vi "Read Core OOB RX.vi"(8 "error in (no error)":errorcluster, 11 "CIFCorePlugin in":refnum<class "CIFCorePlugin.lvclass">) -> (0 "error out":errorcluster, 3 "CIFCorePlugin out":refnum<class "CIFCorePlugin.lvclass">)   [LabVIEW 2021, in "CIFCorePlugin.lvclass"]
uses:
  CIFCorePlugin.lvclass
  Typedef/gRPC to Main Command Payload.ctl
  Typedef/gRPC to Main Commands.ctl
  <vilib>/CIF Foundation/CIF CIPC/TypeDefs/Read Configuration.ctl
  <vilib>/CIF Foundation/CIF CIPC/TypeDefs/Read Position.ctl
  CIFCorePlugin.lvclass/CIFCorePlugin.ctl
  Common/Typedef/Plugin State.ctl
  Typedef/Energized States.ctl
  <vilib>/CIF Foundation/CIF Channels Core/ChannelCommon/typedef/New FIFO Instance Response.ctl
  Channels/CIFChannelMng/CIFChannelMng.lvclass/CIFChannelMng.ctl
  <vilib>/CIF Foundation/CIF Channels Core/CIFChannels/CIFChannels.lvclass/CIFChannels.ctl
  a31a91a9-4107-4750-8e0d-44486e9a3a34.vi
  Channels/CIFChannelMng/Core/Send Channel List Update.vi/463ebf4c-8748-40f9-8ad3-9e61c16a01a6.vi
  Channels/CIFChannelMng/Utilities/Get Channel Index by Name.vi
  <vilib>/CIF Foundation/CIF Channels Core/CIFChannels/Accessors/Read Channel State.vi
  <vilib>/CIF Foundation/CIF Channels Core/CIFChannels/Accessors/Read Tag Forced.vi
  Channels/CIFChannelMng/SubVIs/Add Error Channel Manager.vi
  Channels/CIFChannelMng/Core/Send Publisher Instance Return.vi/9db40550-ae0b-4108-a32d-02e81b824dbe.vi
  Channels/CIFChannelMng/SubVIs/Get Original FIFO Channel Name.vi
  <vilib>/CIF Foundation/CIF CIPC/SubVIs/Wait For N Elements Available.vi
  <vilib>/CIF Foundation/CIF CIPC/SubVIs/Check Error.vi
  <vilib>/CIF Foundation/CIF CIPC/SubVIs/Get dll Path.vi
  <vilib>/CIF Foundation/CIF CIPC/SubVIs/Get Element Read Position.vi
  <vilib>/CIF Foundation/CIF CIPC/SubVIs/Set Element Read Position.vi
  <vilib>/CIF Foundation/CIF CIPC/SubVIs/Notify Of New Write.vi
  <vilib>/CIF Foundation/CIF CIPC/SubVIs/Get Element Write Position.vi
  <vilib>/CIF Foundation/CIF Channels Core/ChannelCommon/Utilities/Add Error.vi
  <vilib>/CIF Foundation/CIF Utilities/Errors/Append Error Location.vi
  <vilib>/CIF Foundation/CIF CIPC/SubVIs/Get Element Info Variant.vi
  <vilib>/CIF Foundation/CIF CIPC/SubVIs/Check Error Core.vi
  <vilib>/CIF Foundation/CIF Channels Core/ChannelCommon/Utilities/Add Error Core.vi
  <vilib>/CIF Foundation/CIF Channels Core/CIFChannels/Core/Set Force.vi
  <vilib>/CIF Foundation/CIF Channels Core/CIFChannels/CIFChannels.lvclass
  Channels/CIFChannelMng/CIFChannelMng.lvclass
  <vilib>/CIF Foundation/CIF CIPC/CIF_NI_CIPC.lvlib
  <vilib>/CIF Foundation/CIF Channels Core/ChannelCommon/ChannelCommon.lvlib
  Common/CIFCoreCommon.lvlib
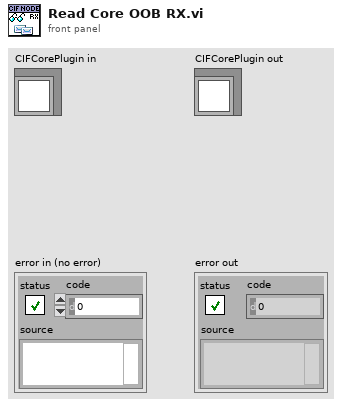
[diagram p1: front panel]
types:
  T1 = typedef "CIFCorePlugin.lvclass/gRPC to Main Command Payload.ctl" = cluster{"OOB_Rx Command":T2, "Array Index":i16}
  T2 = typedef "CIFCorePlugin.lvclass/gRPC to Main Commands.ctl" = enum8{"Start", "Pause", "Stop", "RefreshStats", "UpdateConfig", "Update Clock Map", "Connect Channel", "Force Channel", "Add Publisher Instance", "Remove Publisher Instance", "Prepare"}
  T3 = typedef "CIF_NI_CIPC.lvlib/Read Configuration.ctl" = cluster{"Read Position":T4, "Element Offset":i32, "Prepend Array Size":bool, "Get Read Position":bool}
  T4 = typedef "CIF_NI_CIPC.lvlib/Read Position.ctl" = enum8{"Next", "Newest", "Oldest", "Next Available", "Absolute"}
  T5 = typedef "CIFCoreCommon.lvlib/Plugin State.ctl" = enum8{"Null", "Creating", "Listening", "Running", "CleaningUp", "Destroying", "Prepared", "FTE_Run"}
  T6 = typedef "CIFCorePlugin.lvclass/Energized States.ctl" = enum16{"Listen", "Prepare", "Execute", "Housekeep", "Cleanup", "Destroy"}
  T7 = typedef "ChannelCommon.lvlib/New FIFO Instance Response.ctl" = cluster{"Publisher":string, "Custom Data":u8[]}
  T8 = typedef "Time_CIF_U.lvlib/Clock Conversion Map.ctl" = map{u8, cluster{"Last Reset":i64, "Offset Pair":T9, "Slope":dbl, "1/Slope":dbl}}
  T9 = typedef "Time_CIF_U.lvlib/Timestamp Pair.ctl" = cluster{"System Time":i64, "External Time":i64}
  T10 = typedef "CIFCoreCommon.lvlib/Channel Connection Data.ctl" = cluster{"Publisher Name":string, "Subscriber Name":string, "Connection Data":u8[]}
  T11 = typedef "CIFCoreCommon.lvlib/Channel Force Data.ctl" = cluster{"Channel Name":string, "Force Data":u8[], "Force Active":bool}
  T12 = typedef "CIFCoreCommon.lvlib/FIFO Publisher.ctl" = cluster{"Publisher Name":string, "New FIFO Instance Config":T13}
  T13 = typedef "ChannelCommon.lvlib/New FIFO Instance Configuration.ctl" = cluster{"Backpressure":bool, "Bytes/Message Override":u32, "Messages/FIFO Override":u32, "Custom Data":u8[]}
  T14 = typedef "CIFChannelMng.lvclass/FIFO Publisher Return.ctl" = cluster{"FIFO Instance Config":T7, "error":errorcluster, "Added":bool}
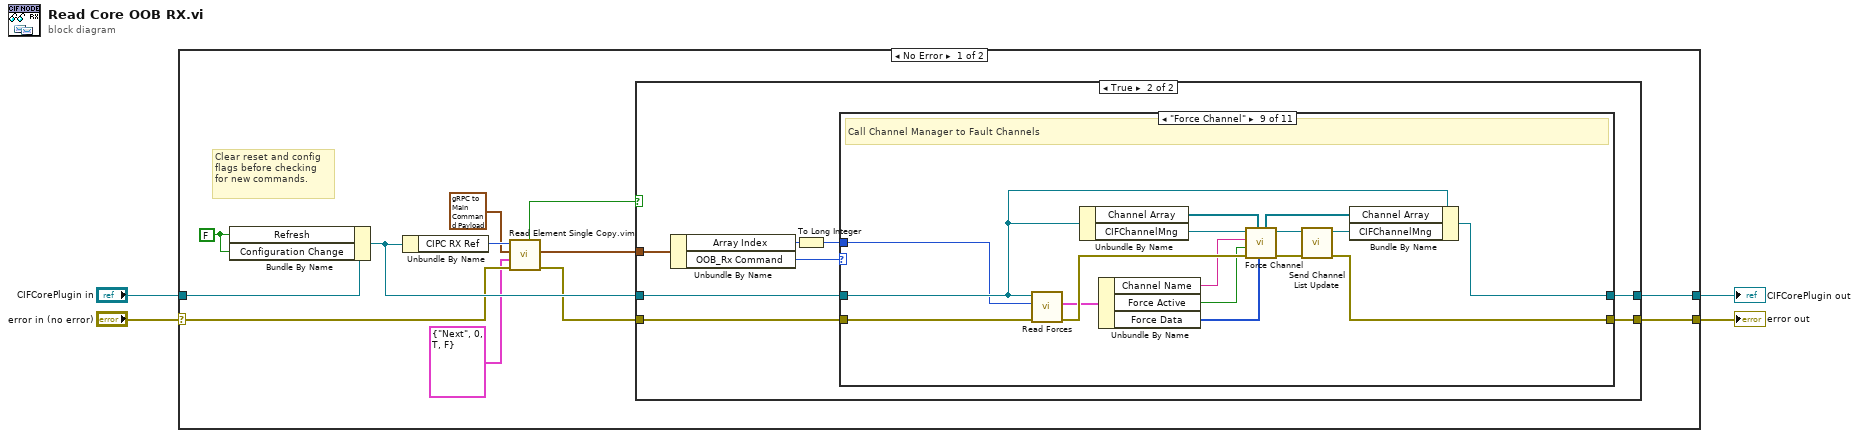
[diagram p0: block diagram]
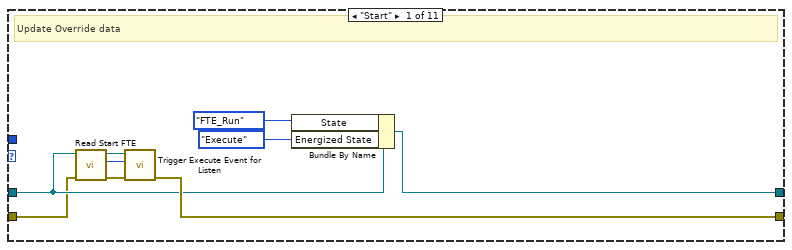
[diagram p3: hidden frame]
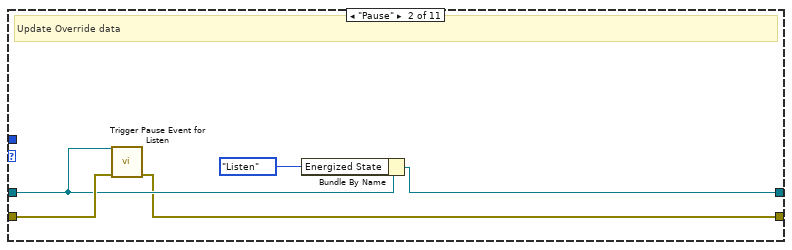
[diagram p4: hidden frame]
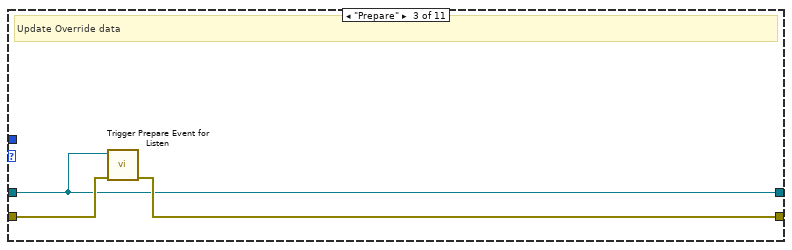
[diagram p5: hidden frame]
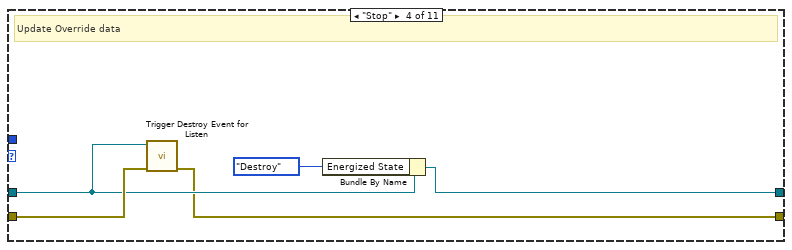
[diagram p6: hidden frame]
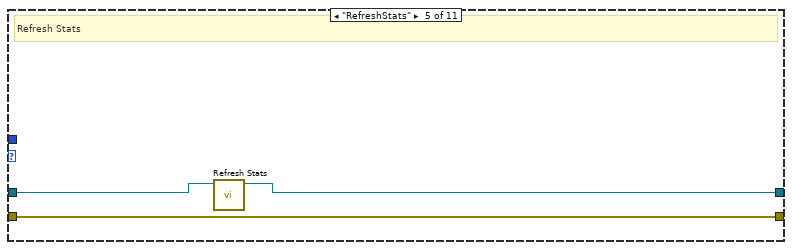
[diagram p7: hidden frame]
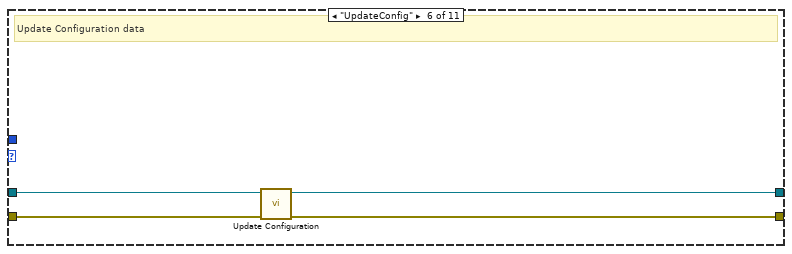
[diagram p8: hidden frame]
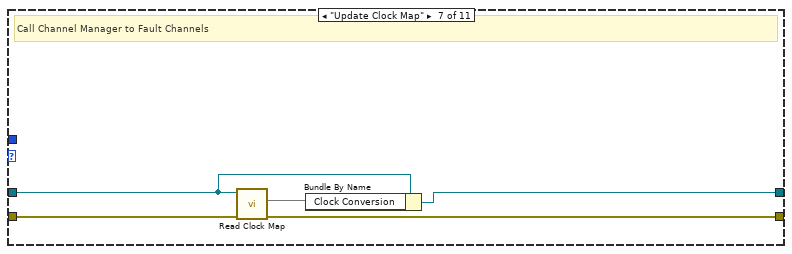
[diagram p9: hidden frame]
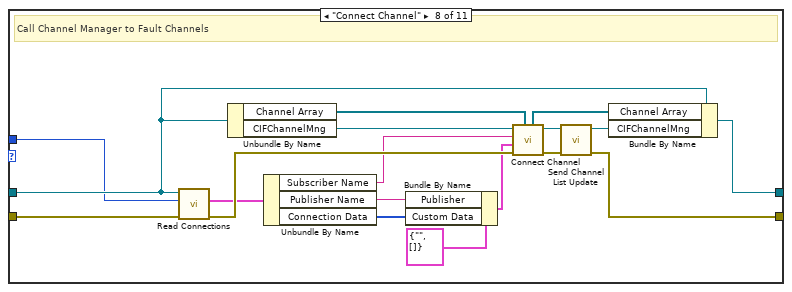
[diagram p10: hidden frame]
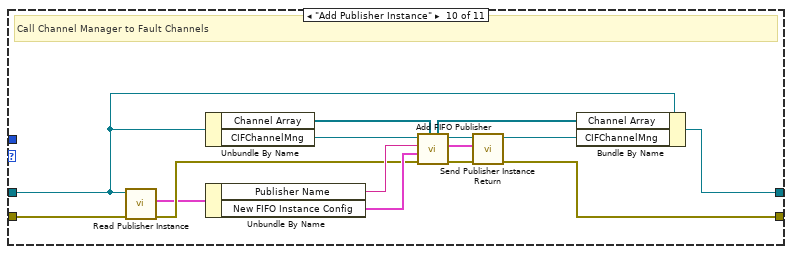
[diagram p11: hidden frame]
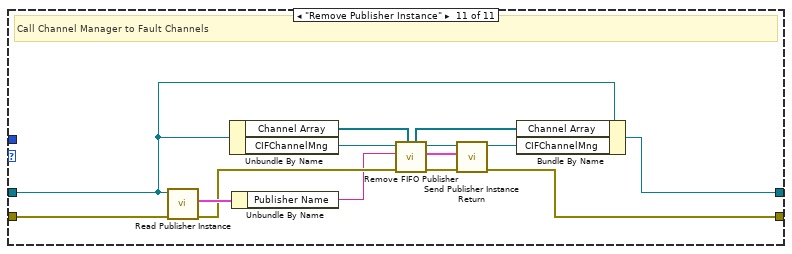
[diagram p12: hidden frame]
diagram:
  n1 = case shown="No Error" "error in (no error)" {
    selector: "error in (no error)" -> [w12 w125]
    tunnel: [w14 w125] -> w1
    tunnel: [w15 w124] -> w2
    tunnel: "CIFCorePlugin in" -> [w16 w124]
    frame No Error {
      w5 = FALSE ("Running Internal Data.Refresh")
      # "Clear reset and config flags before checking for new commands."
      n2 = Bundle By Name(cluster=w16, "Refresh"=w5, "Configuration Change"=w5) -> (w13:refnum<class "CIFCorePlugin.lvclass">)
      n3 = Unbundle By Name(w13) -> ("CIPC RX Ref"=w11:u64)
      n4 = call "Read Element Single Copy.vim"("error in (no error)"=w12, "Read Configuration"=T3 {"Read Position"=enum."Next", "Element Offset"=0, "Prepend Array Size"=TRUE, "Get Read Position"=FALSE}, "Data in"=T1 {"OOB_Rx Command"=enum."Remove Publisher Instance", "Array Index"=0} ("gRCP to Main Command Payload"), "CIPC Reference in"=w11) -> ("error out"=w10:errorcluster, "Data out"=w7:T1, "Success"=w8:bool)  [unwired: 3 in, 2 out]
      n5 = case shown="True" w8 {
        tunnel: w10 -> [w17 w23]
        tunnel: w13 -> [w18 w24]
        tunnel: [w18 w26] -> w15
        tunnel: [w17 w25] -> w14
        tunnel: w7 -> [_ w22]
        frame False {
        }
        frame True {
          n6 = Unbundle By Name(w22) -> ("Array Index"=w20:i16, "OOB_Rx Command"=w21:T2)
          n7 = To Long Integer(number=w20) -> (32bit integer=w19:i32)
          n8 = case shown="\"Force Channel\"" w21 {
            tunnel: w23 -> [w29 w38 w43 w46 w49 w54 w60 w77 w92 w106 w123]
            tunnel: w24 -> [w32 w37 w41 w45 w51 w55 w56 w69 w81 w96 w110]
            tunnel: [w35 w40 w41 w48 w50 w53 w59 w66 w80 w95 w111] -> w26
            tunnel: [w33 w36 w42 w44 w49 w52 w58 w72 w93 w97 w120] -> w25
            tunnel: w19 -> [_ _ _ _ _ _ _ w65 w79 _ _]
            frame "Start" {
              # "Update Override data"
              n9 = call "Read Start FTE.vi"("error in"=w29, "CIFCorePlugin in"=w32) -> ("error out"=w30:errorcluster, "Start FTE"=w28:i64, "CIFCorePlugin out"=w31:refnum<class "CIFCorePlugin.lvclass">)  [unwired: 7 in]
              n10 = call "Trigger Execute Event for Listen.vi"("error in (no error)"=w30, "FTE"=w28, "CIFCorePlugin in"=w31) -> ("error out"=w33:errorcluster)  [unwired: 8 in]
              n11 = Bundle By Name(cluster=w32, "State"=Plugin_State."FTE_Run" ("Main to gRPC Data.Status.State"), "Energized State"=Energized_States."Execute" ("Energized States in")) -> (w35:refnum<class "CIFCorePlugin.lvclass">)
            }
            frame "Pause" {
              # "Update Override data"
              n12 = call "Trigger Pause Event for Listen.vi"("error in (no error)"=w38, "CIFCorePlugin in"=w37) -> ("error out"=w36:errorcluster)  [unwired: 9 in]
              n13 = Bundle By Name(cluster=w37, "Energized State"=Energized_States."Listen" ("Energized States in")) -> (w40:refnum<class "CIFCorePlugin.lvclass">)
            }
            frame "Prepare" {
              # "Update Override data"
              n14 = call "Trigger Prepare Event for Listen.vi"("error in (no error)"=w43, "CIFCorePlugin in"=w41) -> ("error out"=w42:errorcluster)  [unwired: 9 in]
            }
            frame "Stop" {
              # "Update Override data"
              n15 = call "Trigger Destroy Event for Listen.vi"("error in (no error)"=w46, "CIFCorePlugin in"=w45) -> ("error out"=w44:errorcluster)  [unwired: 9 in]
              n16 = Bundle By Name(cluster=w45, "Energized State"=Energized_States."Destroy" ("Energized States in")) -> (w48:refnum<class "CIFCorePlugin.lvclass">)
            }
            frame "RefreshStats" {
              # "Refresh Stats"
              n17 = call "Refresh Stats.vi"("CIFCorePlugin in"=w51) -> ("CIFCorePlugin out"=w50:refnum<class "CIFCorePlugin.lvclass">)  [unwired: 10 in]
            }
            frame "UpdateConfig" {
              # "Update Configuration data"
              n18 = call-dynamic "Update Configuration.vi"("error in (no error)"=w54, "CIFTemplateNode in"=w55) -> ("error out"=w52:errorcluster, "CIFTemplateNode out"=w53:refnum<class "CIFCorePlugin.lvclass">)  [unwired: 8 in]
            }
            frame "Update Clock Map" {
              # "Call Channel Manager to Fault Channels"
              n19 = call "Read Clock Map.vi"("error in"=w60, "CIFCorePlugin in"=w56) -> ("error out"=w58:errorcluster, "Clock Conversion"=w57:T8)  [unwired: 7 in, 1 out]
              n20 = Bundle By Name(cluster=w56, "Clock Conversion"=w57) -> (w59:refnum<class "CIFCorePlugin.lvclass">)
            }
            frame "Connect Channel" {
              # "Call Channel Manager to Fault Channels"
              n21 = call "Read Connections.vi"("error in"=w77, "index"=w65, "CIFCorePlugin in"=w69) -> ("error out"=w73:errorcluster, "Connection"=w67:T10)  [unwired: 6 in, 1 out]
              n22 = Unbundle By Name(w69) -> ("Channel Array"=w71:refnum<class "CIFChannels.lvclass">[], "CIFChannelMng"=w78:refnum<class "CIFChannelMng.lvclass">)
              n23 = Unbundle By Name(w67) -> ("Subscriber Name"=w68:string, "Publisher Name"=w63:string, "Connection Data"=w62:u8[])
              n24 = Bundle By Name(cluster=T7 {"Publisher"="", "Custom Data"=[]} ("Connection"), "Publisher"=w63, "Custom Data"=w62) -> (w61:T7)
              n25 = call "Connect Channel.vi"("Channel Array in"=w71, "error in (no error)"=w73, "Connection"=w61, "Subscriber Name"=w68, "CIFChannelMng in"=w78) -> ("error out"=w75:errorcluster, "CIFChannelMng out"=w76:refnum<class "CIFChannelMng.lvclass">, "Channel Array out"=w70:refnum<class "CIFChannels.lvclass">[])  [unwired: 3 in, 1 out]
              n26 = call "Send Channel List Update.vi"("error in (no error)"=w75, "CIFChannelMng in"=w76) -> ("error out"=w72:errorcluster, "CIFChannelMng out"=w74:refnum<class "CIFChannelMng.lvclass">)  [unwired: 8 in]
              n27 = Bundle By Name(cluster=w69, "Channel Array"=w70, "CIFChannelMng"=w74) -> (w66:refnum<class "CIFCorePlugin.lvclass">)
            }
            frame "Force Channel" {
              # "Call Channel Manager to Fault Channels"
              n28 = call "Read Forces.vi"("error in"=w92, "index"=w79, "CIFCorePlugin in"=w81) -> ("error out"=w90:errorcluster, "Force"=w82:T11)  [unwired: 6 in, 1 out]
              n29 = Unbundle By Name(w81) -> ("Channel Array"=w87:refnum<class "CIFChannels.lvclass">[], "CIFChannelMng"=w91:refnum<class "CIFChannelMng.lvclass">)
              n30 = Unbundle By Name(w82) -> ("Channel Name"=w85:string, "Force Active"=w84:bool, "Force Data"=w83:u8[])
              n31 = call "Force Channel.vi"("Force Data"=w83, "Channel Array in"=w87, "error in (no error)"=w90, "Force Active"=w84, "Channel Name"=w85, "CIFChannelMng in"=w91) -> ("error out"=w89:errorcluster, "CIFChannelMng out"=w88:refnum<class "CIFChannelMng.lvclass">, "Channel Array out"=w86:refnum<class "CIFChannels.lvclass">[])  [unwired: 2 in, 1 out]
              n32 = call "Send Channel List Update.vi"("error in (no error)"=w89, "CIFChannelMng in"=w88) -> ("error out"=w93:errorcluster, "CIFChannelMng out"=w94:refnum<class "CIFChannelMng.lvclass">)  [unwired: 8 in]
              n33 = Bundle By Name(cluster=w81, "Channel Array"=w86, "CIFChannelMng"=w94) -> (w80:refnum<class "CIFCorePlugin.lvclass">)
            }
            frame "Add Publisher Instance" {
              # "Call Channel Manager to Fault Channels"
              n34 = call "Read Publisher Instance.vi"("error in"=w106, "CIFCorePlugin in"=w96) -> ("error out"=w105:errorcluster, "Publisher Instance"=w104:T12)  [unwired: 7 in, 1 out]
              n35 = Unbundle By Name(w96) -> ("Channel Array"=w100:refnum<class "CIFChannels.lvclass">[], "CIFChannelMng"=w109:refnum<class "CIFChannelMng.lvclass">)
              n36 = Unbundle By Name(w104) -> ("Publisher Name"=w108:string, "New FIFO Instance Config"=w107:T13)
              n37 = call "Add FIFO Publisher.vi"("Channel Array in"=w100, "error in (no error)"=w105, "New FIFO Instance Config"=w107, "Channel Name"=w108, "CIFChannelMng in"=w109) -> ("error out"=w102:errorcluster, "FIFO Publisher"=w101:T14, "CIFChannelMng out"=w103:refnum<class "CIFChannelMng.lvclass">, "Channel Array out"=w99:refnum<class "CIFChannels.lvclass">[])  [unwired: 2 in, 1 out]
              n38 = call "Send Publisher Instance Return.vi"("error in (no error)"=w102, "Publisher Instance"=w101, "CIFChannelMng in"=w103) -> ("error out"=w97:errorcluster, "CIFChannelMng out"=w98:refnum<class "CIFChannelMng.lvclass">)  [unwired: 7 in]
              n39 = Bundle By Name(cluster=w96, "Channel Array"=w99, "CIFChannelMng"=w98) -> (w95:refnum<class "CIFCorePlugin.lvclass">)
            }
            frame "Remove Publisher Instance" {
              # "Call Channel Manager to Fault Channels"
              n40 = call "Read Publisher Instance.vi"("error in"=w123, "CIFCorePlugin in"=w110) -> ("error out"=w118:errorcluster, "Publisher Instance"=w122:T12)  [unwired: 7 in, 1 out]
              n41 = Unbundle By Name(w110) -> ("Channel Array"=w113:refnum<class "CIFChannels.lvclass">[], "CIFChannelMng"=w119:refnum<class "CIFChannelMng.lvclass">)
              n42 = Unbundle By Name(w122) -> ("Publisher Name"=w117:string)
              n43 = call "Remove FIFO Publisher.vi"("Channel Array in"=w113, "error in (no error)"=w118, "Channel Name"=w117, "CIFChannelMng in"=w119) -> ("error out"=w116:errorcluster, "FIFO Publisher"=w115:T14, "CIFChannelMng out"=w114:refnum<class "CIFChannelMng.lvclass">, "Channel Array out"=w112:refnum<class "CIFChannels.lvclass">[])  [unwired: 3 in, 1 out]
              n44 = call "Send Publisher Instance Return.vi"("error in (no error)"=w116, "Publisher Instance"=w115, "CIFChannelMng in"=w114) -> ("error out"=w120:errorcluster, "CIFChannelMng out"=w121:refnum<class "CIFChannelMng.lvclass">)  [unwired: 7 in]
              n45 = Bundle By Name(cluster=w110, "Channel Array"=w112, "CIFChannelMng"=w121) -> (w111:refnum<class "CIFCorePlugin.lvclass">)
            }
          }
        }
      }
    }
    frame Error {
    }
  }
  "error out" <- w1
  "CIFCorePlugin out" <- w2
